vi "ANC_stripped.vi"() -> ()   [LabVIEW 2019]
uses:
  <vilib>/sound2/lvsound2.llb/Sound Data Format.ctl
  <vilib>/sound2/lvsound2.llb/Sampling Mode.ctl
  <vilib>/sound2/lvsound2.llb/Sound Output Write (DBL Single).vi
  Dynamic-Link Library.dll
panel:
  in  "Case Choice":u16(ring) items=["Case 1: Feedforward", "Case 2: Feedback/Hybrid"]
  in  "mu (step size)":dbl min=0.0 max=0.1 step=0.0001
  in  "UI Stop":bool
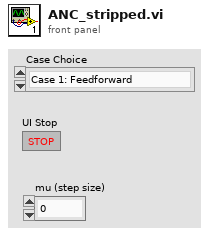
[diagram p1: front panel]
types:
  T1 = typedef "Sampling Mode.ctl" = i32
  T2 = typedef "Sound Data Format.ctl" = cluster{"sample rate (S/s)":dbl, "number of channels":i32, "bits per sample":i32}
  T3 = typedef "Sound Output Task ID.ctl" = u32
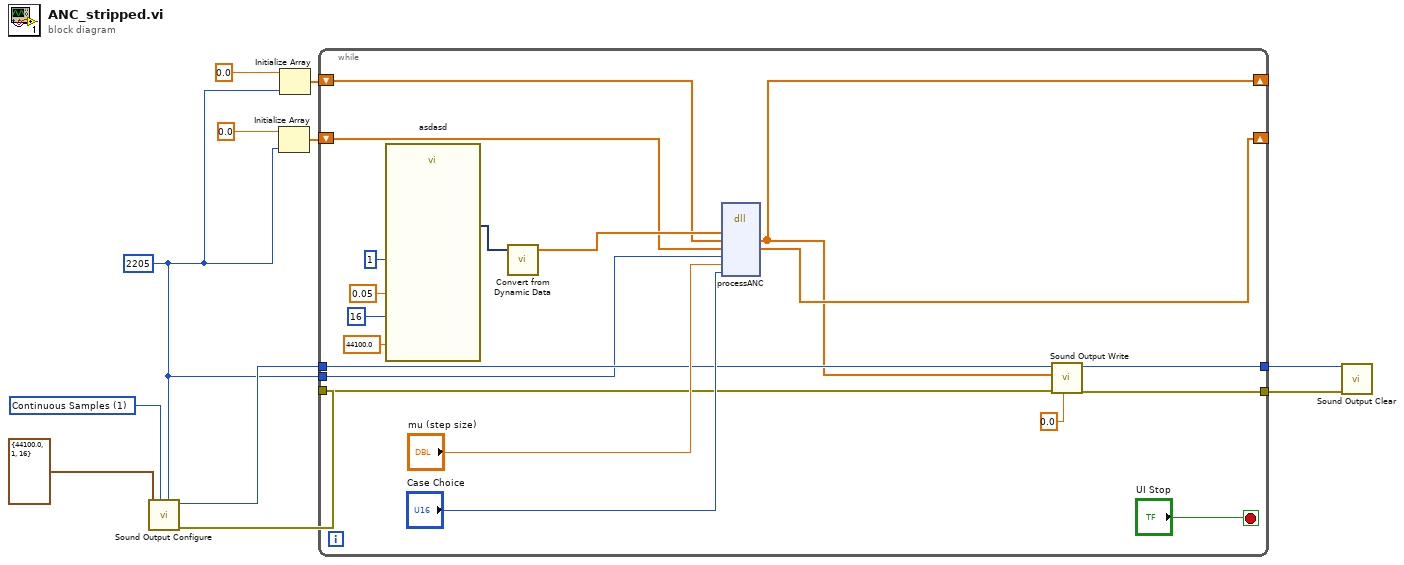
[diagram p0: block diagram]
diagram:
  w8 = T1 1 items=["Finite Samples", "Continuous Samples"] ("sample mode")
  w1 = 2205 ("number of samples/ch")
  n1 = call <vilib>:"Sound Output Configure.vi"("number of samples/ch"=w1, "sample mode"=w8, "sound format"=T2 {"sample rate (S/s)"=44100.0, "number of channels"=1, "bits per sample"=16}) -> ("error out"=w6:errorcluster, "task ID"=w7:T3)  [unwired: 7 in]
  n2 = Initialize Array(0.0 ("element"), w1) -> (w2:dbl[])
  n3 = Initialize Array(0.0 ("element"), w1) -> (w10:dbl[])
  n4 = while {
    shift-right: [w13] -> _
    shift-left: w10 -> [w22]
    tunnel: w7 -> [w27]
    tunnel: w6 -> [w26]
    tunnel: [w25] -> w5
    tunnel: [w24] -> w4
    shift-right: [w20] -> _
    shift-left: w2 -> [w21]
    tunnel: w1 -> [w12]
    stop <- "UI Stop" stop-if-true
    n5 = call "asdasd.vi"("Duration (s)"=0.05, "Sample rate (Hz)"=44100.0, "#Channels"=1, "Resolution (bits)"=16) -> ("Data"=w19:dynamicdata)  [unwired: 14 in, 1 out]
    n6 = call "Convert from Dynamic Data"("Dynamic Data Type"=w19) -> ("Array"=w23:dbl[])  [unwired: 3 in]
    n7 = dll-call lib="C:/Users/akdag/Desktop/EE433/433_Project/Final/EE433_ANC_Engine/EE433_ANC_Engine/Dynamic-Link Library.dll" fn="processANC"("mic1"=w23, "output"=w22, "clean_error"=w21, "frameSize"=w12, "mu"="mu (step size)", "caseSelection"="Case Choice") -> ("output"=w13:dbl[], "clean_error"=w20:dbl[])  [unwired: 8 in, 2 out]
    n8 = call-poly <vilib>:"Sound Output Write.vi"("timeout (sec)"=0.0, "error in (no error)"=w26, "data"=w13, "task ID"=w27) -> ("error out"=w24:errorcluster, "task ID out"=w25:T3)  [unwired: 6 in]
  }
  n9 = call <vilib>:"Sound Output Clear.vi"("error in (no error)"=w4, "task ID"=w5) -> ()  [unwired: 9 in, 1 out]
